vi "checkBeginSimpleBallPlacementAllyPlay.vi"(8 "error in (no error)":errorcluster, 10 "Game":refnum<class "Game.lvclass">, 11 "SimpleBallPlacementAllyPlay in":refnum<class "SimpleBallPlacementAllyPlay.lvclass">) -> (0 "error out":errorcluster, 2 "begin":bool, 3 "SimpleBallPlacementAllyPlay out":refnum<class "SimpleBallPlacementAllyPlay.lvclass">)   [LabVIEW 2023, in "SimpleBallPlacementAllyPlay.lvclass"]
uses:
  SimpleBallPlacementAllyPlay.lvclass
  Game_class/Game.lvclass
  Referee_class/command_interpreted.ctl
  Game_class/Game.lvclass/Game.ctl
  Object_class/Object.lvclass/Object.ctl
  Referee_class/Referee.lvclass/Referee.ctl
  Game_class/Read Referee.vi
  Game_class/Read BallRef.vi
  Object_class/Read position(x,y).vi
  Referee_class/Read command_interpreted.vi
  Ball_class/Ball.lvclass
  C:/Users/lucio/Desktop/roboime/SSL_AI/Object_class/Object.lvclass
  Referee_class/Referee.lvclass
  Utilities_class/Utilities.lvclass
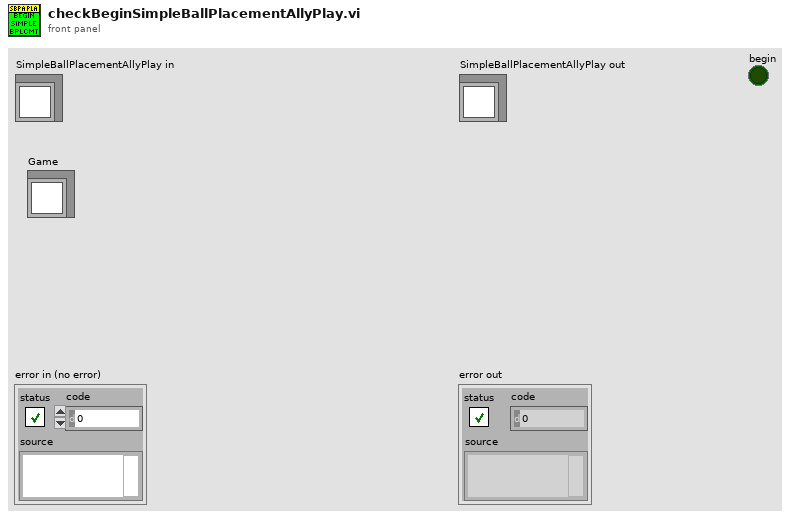
[diagram p1: front panel]
types:
  T1 = typedef "command_interpreted.ctl" = enum16{"Goal Ally", "Goal Enemy", "Ball Placement Enemy", "Ball Placement Ally", "Normal Half Time", "Extra Time  Break", "Extra Half Time", "None", "Post Game", "PKA Normal Start", "Prepare Kickoff Ally", "PKE Normal Start", "Prepare Kickoff Enemy", "Force Start", "Halt", "Timeout", "Prepare Penalty Ally", "Prepare Penalty Enemy", "PPA NormalStart", "PPE Normal Start", "Indirect Free Ally", "Direct Free Enemy", "Direct Free Ally", "Indirect Free Enemy", "Stop"}
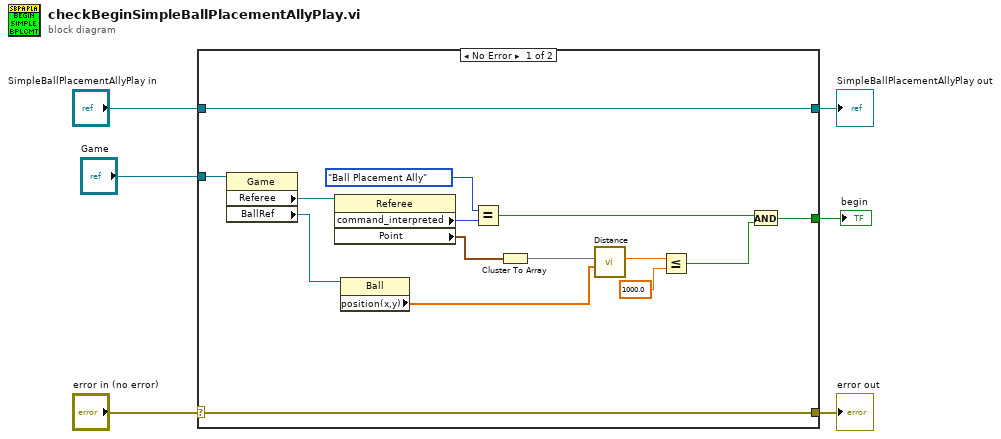
[diagram p0: block diagram]
diagram:
  n1 = case shown="No Error" "error in (no error)" {
    selector: "error in (no error)" -> [w20 w23]
    tunnel: [w20 w23] -> w5
    tunnel: [w21 w22] -> w3
    tunnel: "SimpleBallPlacementAllyPlay in" -> [w21 w22]
    tunnel: "Game" -> [w19 _]
    tunnel: [w16 _] -> w1
    frame No Error {
      n2 = property class="Game"(reference=w19) -> ("Referee"=w18:refnum<class "Referee.lvclass">, "BallRef"=w13:refnum<class "Ball.lvclass">)  [unwired: 1 in, 2 out]
      n3 = property class="Referee"(reference=w18) -> ("command_interpreted"=w14:T1, "Point"=w8:cluster{"x":sgl, "y":sgl})  [unwired: 1 in, 2 out]
      n4 = property class="Ball"(reference=w13) -> ("position(x,y)"=w12:dbl[])  [unwired: 1 in, 2 out]
      n5 = Equal?(x=command_interpreted."Ball Placement Ally" ("y"), y=w14) -> (x = y?=w17:bool)
      n6 = Cluster To Array(cluster=w8) -> (array=w7:sgl[])
      n7 = call "Distance.vi"("P1"=w12, "P2"=w7) -> ("Distance"=w11:dbl)  [unwired: 7 in, 2 out]
      n8 = Less Or Equal?(x=w11, y=1000.0) -> (x <= y?=w9:bool)
      n9 = And(x=w17, y=w9) -> (x .and. y?=w16:bool)
    }
    frame Error {
    }
  }
  "error out" <- w5
  "SimpleBallPlacementAllyPlay out" <- w3
  "begin" <- w1
